vi "Interpolate data.vi"(6 "Interpolation Direction":enum16{"Horizontal", "Vertical", "2-D"}(ring), 7 "Draw Area Size":cluster{"Width":u32, "Height":u32}, 8 "error in":errorcluster, 11 "Data":dbl[][](array[numeric])=array32x1250[40000 elements]) -> (0 "error out":errorcluster, 3 "Resampled Data":dbl[][](array[numeric]))   [LabVIEW 2009]
doc: "This VI interpolates or decimates 2-D data sets to fit them into a specified grid. The VI can be used to interpolate horizontally, vertically, or both, as specified by the Interpolation Direction control."
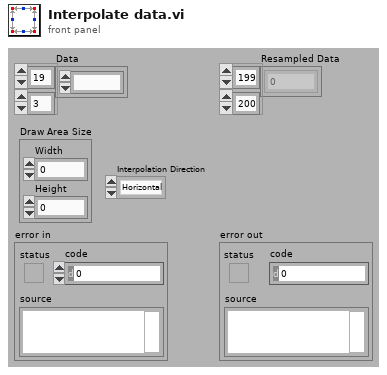
[diagram p1: front panel]
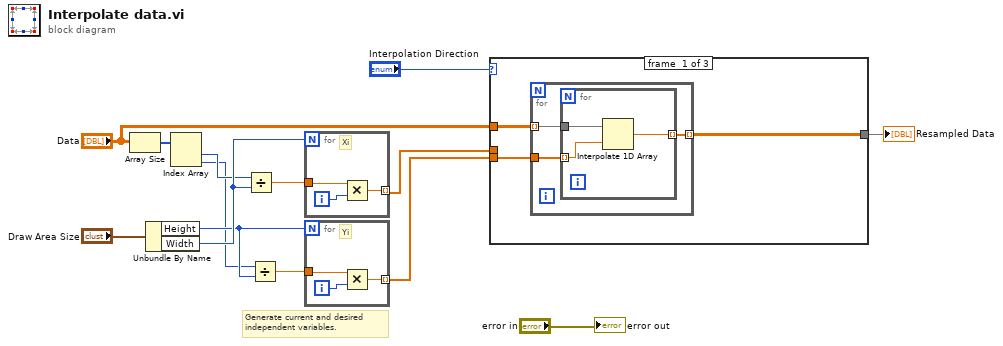
[diagram p0: block diagram]
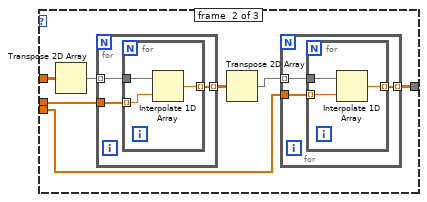
[diagram p2: hidden frame]
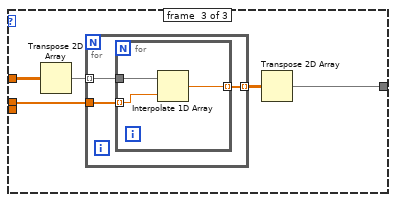
[diagram p3: hidden frame]
diagram:
  # "Generate current and desired\nindependent variables."
  n1 = Array Size(array="Data") -> (size(s)=w14:i32[])
  n2 = Unbundle By Name("Draw Area Size") -> ("Height"=w10:u32, "Width"=w12:u32)
  n3 = Index Array(array=w14) -> (element #1=w8:i32, element #2=w7:i32)  [unwired: 2 in]
  n4 = Divide(x=w8, y=w12) -> (x/y=w11:dbl)
  n5 = Divide(x=w7, y=w10) -> (x/y=w1:dbl)
  n6 = for {
    N: w12 -> [_]
    tunnel: w11 -> [w17]
    tunnel: [w16] -> w6 mode=indexing
    i -> [w15]
    # "Xi"
    n7 = Multiply(x=w17, y=w15) -> (x*y=w16:dbl)
  }
  n8 = for {
    N: w10 -> [_]
    tunnel: w1 -> [w18]
    tunnel: [w20] -> w5 mode=indexing
    i -> [w19]
    # "Yi"
    n9 = Multiply(x=w18, y=w19) -> (x*y=w20:dbl)
  }
  n10 = case shown="\"2-D\"" "Interpolation Direction" {
    tunnel: w6 -> [_ w30 w53]
    tunnel: w5 -> [w22 w36 _]
    tunnel: "Data" -> [w23 w32 w52]
    tunnel: [w21 w35 w49] -> w2
    frame #0 {
      n11 = for {
        tunnel: w23 -> [w25] mode=indexing
        tunnel: w22 -> [w26]
        tunnel: [w24] -> w21 mode=indexing
        n12 = for {
          tunnel: w26 -> [w28] mode=indexing
          tunnel: w25 -> [w29]
          tunnel: [w27] -> w24 mode=indexing
          n13 = Interpolate 1D Array(1:w28, 2:w29) -> (0:w27:dbl)
        }
      }
    }
    frame #1 {
      n14 = Transpose 2D Array(2D array=w32) -> (transposed array=w31:dbl[][])
      n15 = for {
        tunnel: w31 -> [w44] mode=indexing
        tunnel: w30 -> [w45]
        tunnel: [w43] -> w34 mode=indexing
        n16 = for {
          tunnel: w45 -> [w47] mode=indexing
          tunnel: w44 -> [w48]
          tunnel: [w46] -> w43 mode=indexing
          n17 = Interpolate 1D Array(1:w47, 2:w48) -> (0:w46:dbl)
        }
      }
      n18 = Transpose 2D Array(2D array=w34) -> (transposed array=w33:dbl[][])
      n19 = for {
        tunnel: w33 -> [w38] mode=indexing
        tunnel: w36 -> [w39]
        tunnel: [w37] -> w35 mode=indexing
        n20 = for {
          tunnel: w39 -> [w41] mode=indexing
          tunnel: w38 -> [w42]
          tunnel: [w40] -> w37 mode=indexing
          n21 = Interpolate 1D Array(1:w41, 2:w42) -> (0:w40:dbl)
        }
      }
    }
    frame #2 {
      n22 = Transpose 2D Array(2D array=w52) -> (transposed array=w51:dbl[][])
      n23 = for {
        tunnel: w51 -> [w55] mode=indexing
        tunnel: w53 -> [w56]
        tunnel: [w54] -> w50 mode=indexing
        n24 = for {
          tunnel: w56 -> [w58] mode=indexing
          tunnel: w55 -> [w59]
          tunnel: [w57] -> w54 mode=indexing
          n25 = Interpolate 1D Array(1:w58, 2:w59) -> (0:w57:dbl)
        }
      }
      n26 = Transpose 2D Array(2D array=w50) -> (transposed array=w49:dbl[][])
    }
  }
  "Resampled Data" <- w2
  "error out" <- "error in"
